vi "FileErrorHandler.vi"(8 "error in (no error)":errorcluster, 11 "Qbus in":refnum<class "Qbus.lvclass">) -> (0 "error out":errorcluster, 3 "Qbus out":refnum<class "Qbus.lvclass">)   [LabVIEW 2017, in "ServerComm.lvlib"]
uses:
  <vilib>/addons/InsightCM/Devices/Shared/Common/ServerComm/ServerComm.lvlib
  <vilib>/addons/Qbus/Qbus.lvclass
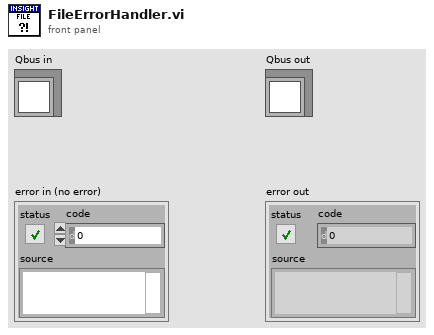
[diagram p1: front panel]
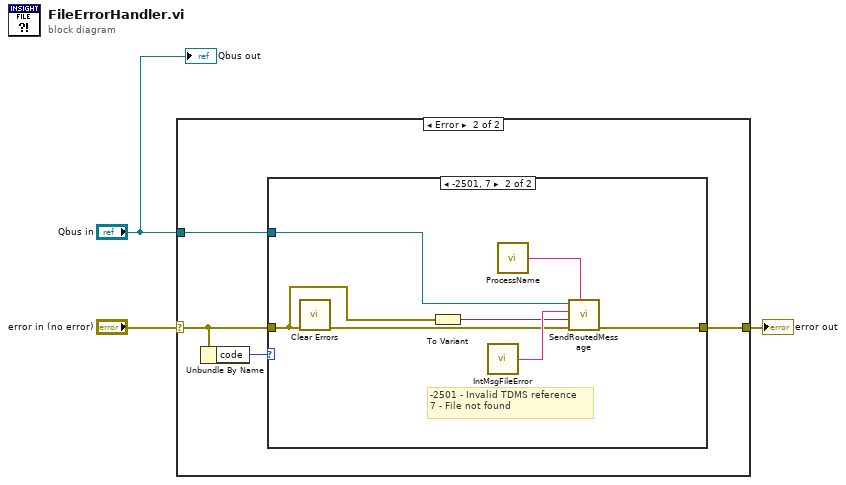
[diagram p0: block diagram]
diagram:
  n1 = case shown="Error" "error in (no error)" {
    selector: "error in (no error)" -> [w4 w7]
    tunnel: [w4 w6] -> w2
    tunnel: "Qbus in" -> [_ w5]
    frame No Error {
    }
    frame Error {
      n2 = Unbundle By Name(w7) -> ("code"=w8:i32)
      n3 = case shown="-2501, 7" w8 {
        tunnel: w7 -> [w9 w11]
        tunnel: [w9 w16] -> w6
        tunnel: w5 -> [_ w12]
        frame Default {
        }
        frame -2501, 7 {
          # "-2501 - Invalid TDMS reference\n7 - File not found"
          n4 = call <vilib>:"Clear Errors.vi"("error in (no error)"=w11) -> ("error out"=w13:errorcluster)  [unwired: 5 in, 1 out]
          n5 = To Variant(anything=w11) -> (Variant=w10:variant)
          n6 = call <vilib>:"IntMsgFileError.vi"() -> ("message name"=w14:string)  [unwired: 5 in]
          n7 = call <vilib>:"ProcessName.vi"() -> ("process name"=w15:string)  [unwired: 5 in]
          n8 = call <vilib>:"SendRoutedMessage.vi"("listener process"=w15, "error in (no error)"=w13, "message value"=w10, "message name"=w14, "Qbus in"=w12) -> ("error in (no error)"=w16:errorcluster)  [unwired: 5 in, 1 out]
        }
      }
    }
  }
  "error out" <- w2
  "Qbus out" <- "Qbus in"
